vi "Serial.vi"(0 "mbed_LVLibrary.lvlib:mbed.lvclass":refnum<class "mbed.lvclass">, 5 "Tx Pin":string, 7 "Rx Pin":string, 9 "Existing Obj Name":string, 11 "error in (no error)":errorcluster) -> (4 "Serial.lvclass 2":refnum<class "Serial.lvclass">, 10 "Assigned Name":string, 15 "error out":errorcluster)   [LabVIEW 2011, in "mbed_LVLibrary.lvlib" / "Serial.lvclass"]
doc: "Creates a Serial port on the mbed. Takes either the tx and rx pins as strings eg (\"p13\" and \"p14\") or the name of an existing serial object on mbed."
uses:
  Serial.lvclass
  Transport Mechanisms/mbed/mbed.lvclass
  Serial.lvclass/Serial.ctl
  <vilib>/regexp/Match Regular Expression.xnode
panel:
  in  "Serial.lvclass":refnum<class "Serial.lvclass">
  # "This is the constructor for a new Digital Out"
  # "Takes an mbed class (which contains the transport method)\n and puts it as a memeber of the Digital Out class\nIt also either ties an existing instance on mbed or creates one"
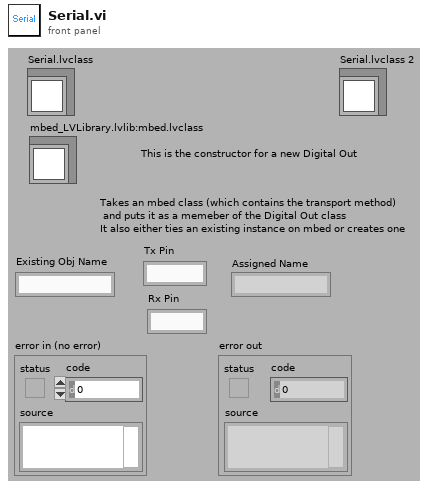
[diagram p1: front panel]
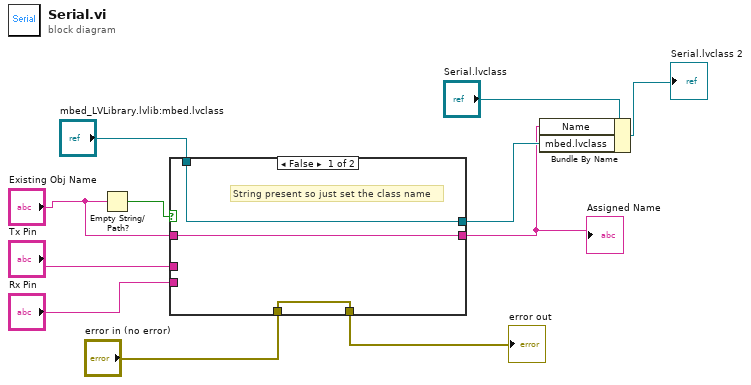
[diagram p0: block diagram]
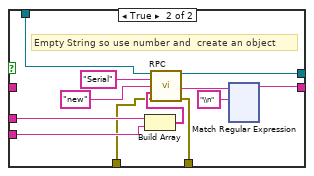
[diagram p2: hidden frame]
diagram:
  n1 = Empty String/Path?(string/path="Existing Obj Name") -> (empty?=w8:bool)
  n2 = case shown="False" w8 {
    tunnel: "Existing Obj Name" -> [w14 _]
    tunnel: [w14 w22] -> w9
    tunnel: "mbed_LVLibrary.lvlib:mbed.lvclass" -> [w13 w26]
    tunnel: [w13 w23] -> w10
    tunnel: "Tx Pin" -> [_ w18]
    tunnel: "Rx Pin" -> [_ w17]
    tunnel: "error in (no error)" -> [w12 w16]
    tunnel: [w12 w15] -> w2
    frame False {
      # "String present so just set the class name"
    }
    frame True {
      # "Empty String so use number and  create an object"
      n3 = Build Array(w18, w17) -> (w19:string[])
      n4 = call-dynamic "RPC.vi"("mbed in"=w26, "Name"="Serial", "method"="new", "Args"=w19, "error in (no error)"=w16) -> ("mbed out"=w23:refnum<class "mbed.lvclass">, "RPC Result"=w21:string, "error out"=w15:errorcluster)  [unwired: 8 in]
      n5 = xnode "Match Regular Expression"("input string"=w21, "regular expression"="\\n") -> ("before match"=w22:string)  [unwired: 4 in, 4 out]
    }
  }
  "Assigned Name" <- w9
  "error out" <- w2
  n6 = Bundle By Name(cluster="Serial.lvclass", "Name"=w9, "mbed.lvclass"=w10) -> (→"Serial.lvclass 2":refnum<class "Serial.lvclass">)
